vi "Analysis.vi"(0 "selected path":path, 9 "VI reference":refnum<vi>, 11 "error in (no error)":errorcluster) -> (2 "SPL":dbl, 3 "Interruption Time (Out)":dbl, 4 "error?":bool, 6 "SGP":dbl, 10 "Resistance (Out)":dbl, 13 "Start Flow":dbl format="%0.3f", 14 "End Flow":dbl format="%0.3f", 15 "error out":errorcluster)   [LabVIEW 2013]
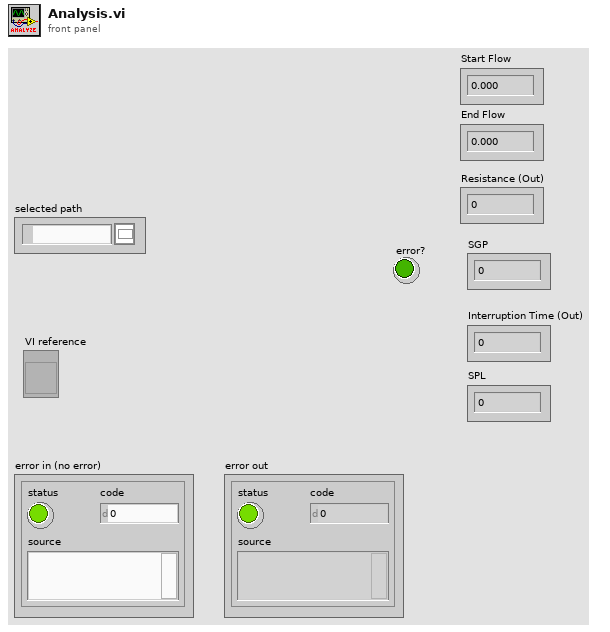
[diagram p1: front panel]
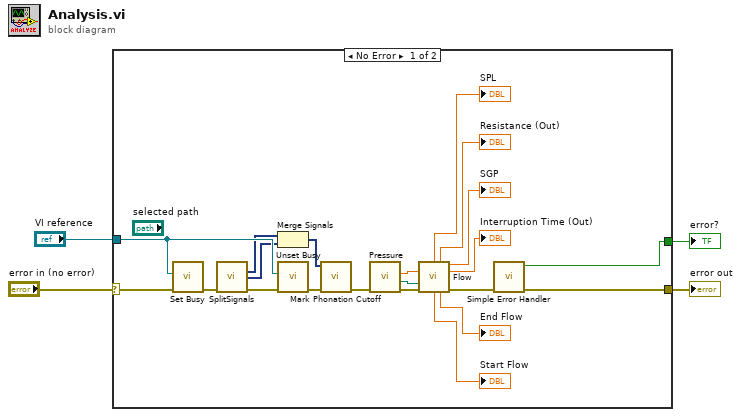
[diagram p0: block diagram]
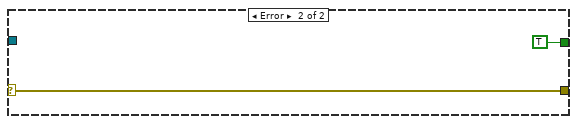
[diagram p2: hidden frame]
diagram:
  n1 = case shown="No Error" "error in (no error)" {
    selector: "error in (no error)" -> [w25 w27]
    tunnel: [w22 w27] -> w4
    tunnel: "VI reference" -> [w24 _]
    tunnel: [w21 TRUE ("error?")] -> w1
    frame No Error {
      n2 = call <vilib>:"Set Busy.vi"("error in (no error)"=w25, "VI reference (current VI)"=w24) -> ("error out"=w7:errorcluster)  [unwired: 8 in, 1 out]
      n3 = call "SplitSignals.vi"("Error In"=w7) -> ("Pressure"=w6:dynamicdata, "Audio"=w5:dynamicdata, "Error Out"=w8:errorcluster)  [unwired: 9 in, 3 out]
      n4 = Merge Signals(w6, w5) -> (w9:dynamicdata)
      n5 = call <vilib>:"Unset Busy.vi"("error in (no error)"=w8, "VI reference (current VI)"=w24) -> ("error out"=w10:errorcluster)  [unwired: 9 in]
      n6 = call "Mark Phonation Cutoff.vi"("Error In"=w10, "Pressure/Audio"=w9) -> ("Error Out"=w11:errorcluster)  [unwired: 6 in, 2 out]
      n7 = call "Pressure.vi"("Error In"=w11) -> ("Error Out"=w20:errorcluster, "File Path Indicator"=w18:path, "Interruption Time"=w19:dbl)  [unwired: 6 in, 1 out]
      n8 = call "Flow.vi"("Interruption Time"=w19, "File Name In"=w18, "Error In"=w20) -> ("SPL"=→"SPL":dbl, "Resistance (Out)"=→"Resistance (Out)":dbl, "SGP"=→"SGP":dbl, "Interruption Time (Out)"=→"Interruption Time (Out)":dbl, "Start Flow"=→"Start Flow":dbl, "End Flow"=→"End Flow":dbl, "Error Out"=w23:errorcluster)  [unwired: 4 in, 2 out]
      n9 = call <vilib>:"Simple Error Handler.vi"("error in (no error)"=w23) -> ("error?"=w21:bool, "error out"=w22:errorcluster)  [unwired: 4 in, 3 out]
    }
    frame Error {
    }
  }
  "error out" <- w4
  "error?" <- w1
